vi "三个模板特征.vi"(8 "Filename 3":path=path "D:/Desktop/test.lvm" caption="sigma 3", 9 "Filename 2":path=path "D:/Desktop/test.lvm" caption="mu 2", 10 "Filename":path=path "D:/Desktop/test.lvm" caption="pai 2") -> (1 "sigma 4":dbl[][](array[numeric]), 2 "mu 3":dbl[][](array[numeric]), 3 "pai 2":dbl[](array[numeric]))   [LabVIEW 2018]
panel:
  out "error out 3":errorcluster caption="错误输出"
  out "Filename Out 3":path caption="文件名输出"
  out "error out 2":errorcluster caption="错误输出"
  out "Filename Out 2":path caption="文件名输出"
  out "error out":errorcluster caption="错误输出"
  out "Filename Out":path caption="文件名输出"
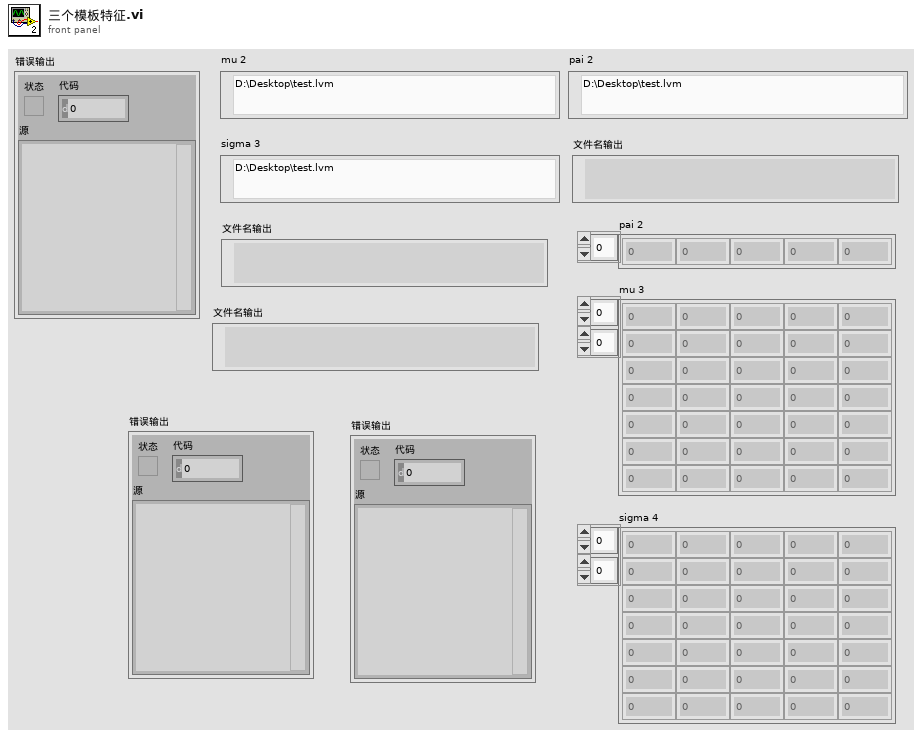
[diagram p1: front panel]
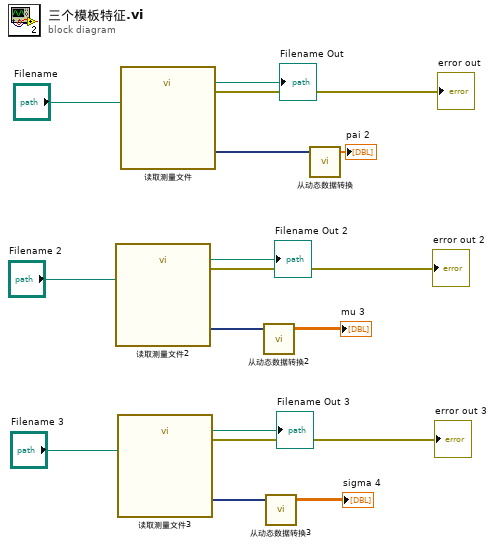
[diagram p0: block diagram]
diagram:
  n1 = call "读取测量文件2"("Filename"="Filename 2") -> ("error out"=→"error out 2":errorcluster, "Filename Out"=→"Filename Out 2":path, "Signals"=w12:dynamicdata)  [unwired: 5 in, 3 out]
  n2 = call "读取测量文件3"("Filename"="Filename 3") -> ("error out"=→"error out 3":errorcluster, "Filename Out"=→"Filename Out 3":path, "Signals"=w7:dynamicdata)  [unwired: 5 in, 3 out]
  n3 = call "读取测量文件"("Filename"="Filename") -> ("error out"=→"error out":errorcluster, "Filename Out"=→"Filename Out":path, "Signals"=w2:dynamicdata)  [unwired: 5 in, 3 out]
  n4 = call "从动态数据转换2"("Dynamic Data Type"=w12) -> ("Array"=→"mu 3":dbl[][])  [unwired: 3 in]
  n5 = call "从动态数据转换3"("Dynamic Data Type"=w7) -> ("Array"=→"sigma 4":dbl[][])  [unwired: 3 in]
  n6 = call "从动态数据转换"("Dynamic Data Type"=w2) -> ("Array"=→"pai 2":dbl[])  [unwired: 3 in]
